vi "setDefaultServer.vi"(8 "error in (no error)":errorcluster, 11 "TcpServer.lvclass":refnum<class "TcpServer.lvclass">) -> (0 "error out":errorcluster, 3 "tcpServer out":refnum<class "TcpServer.lvclass">)   [LabVIEW 2018]
doc: "Help to configure the server to do unit test."
uses:
  src/TcpServer/TcpServer.lvclass
  src/TcpServerTel/typedef/enqueueOptionsTypeDef.ctl
  src/TcpServerTel/TcpServerTel.lvclass
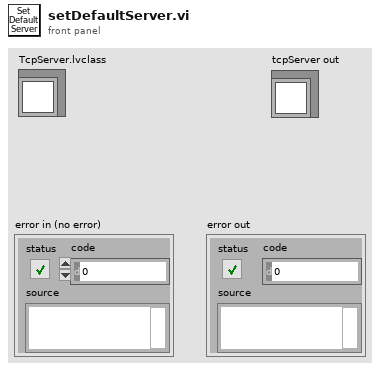
[diagram p1: front panel]
types:
  T1 = typedef "TcpServerTel.lvclass/enqueueOptionsTypeDef.ctl" = enum16{"lossy enqueue", "normal enqueue"}
  T2 = cluster{"cmdServerPort":u16, "telServerPort":u16, "serverTimeout (ms)":i32, "serverBytesToRead":i32, "maxSizeQueueTel":i32, "EnqueueOptions":T1, "timeoutQueueTel (ms)":i32, "tcpClientQueueMaxSize":i32, "timeoutInMs":i32, "runServerTimeoutInMs":i32, "stopServerTimeoutInMs":i32}
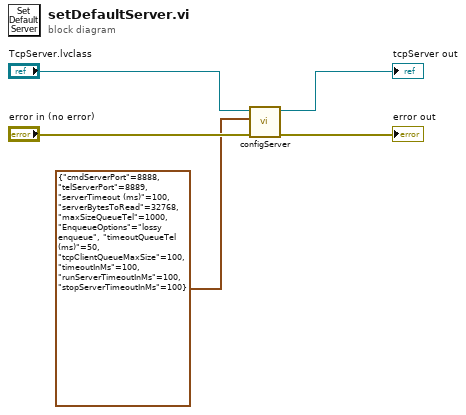
[diagram p0: block diagram]
diagram:
  n1 = call "configServer.vi"("error in (no error)"="error in (no error)", "ServerConfiguration"=T2 {"cmdServerPort"=8888, "telServerPort"=8889, "serverTimeout (ms)"=100, "serverBytesToRead"=32768, "maxSizeQueueTel"=1000, "EnqueueOptions"=enum."lossy enqueue", "timeoutQueueTel (ms)"=50, "tcpClientQueueMaxSize"=100, "timeoutInMs"=100, "runServerTimeoutInMs"=100, "stopServerTimeoutInMs"=100}, "tcpServer in"="TcpServer.lvclass") -> ("error out"=→"error out":errorcluster, "tcpServer out"=→"tcpServer out":refnum<class "TcpServer.lvclass">)  [unwired: 7 in]
